vi "SubVI_SVM_Features.vi"(6 "Sigma":dbl[][](array[numeric]), 7 "MU":dbl[](array[numeric]), 8 "Scale?":bool, 9 "dt":dbl=0.05 format="%#_13g", 10 "window_time":dbl[](array[numeric]), 11 "Sliding_window":dbl[](array[numeric])) -> (1 "min value":dbl, 2 "Features_array":dbl[](array[numeric]), 3 "slope":dbl, 4 "Trap Integrate":dbl format="%0.4f", 5 "Mahibolobis":dbl)   [LabVIEW 2020]
uses:
  <vilib>/Analysis/2dsp.llb/Integral Method.ctl
  <vilib>/Analysis/8numeric.llb/1D Numeric Integration.vi
  <vilib>/Analysis/NI_AALPro.lvlib
panel:
  out "Array":dbl[][](array[numeric])
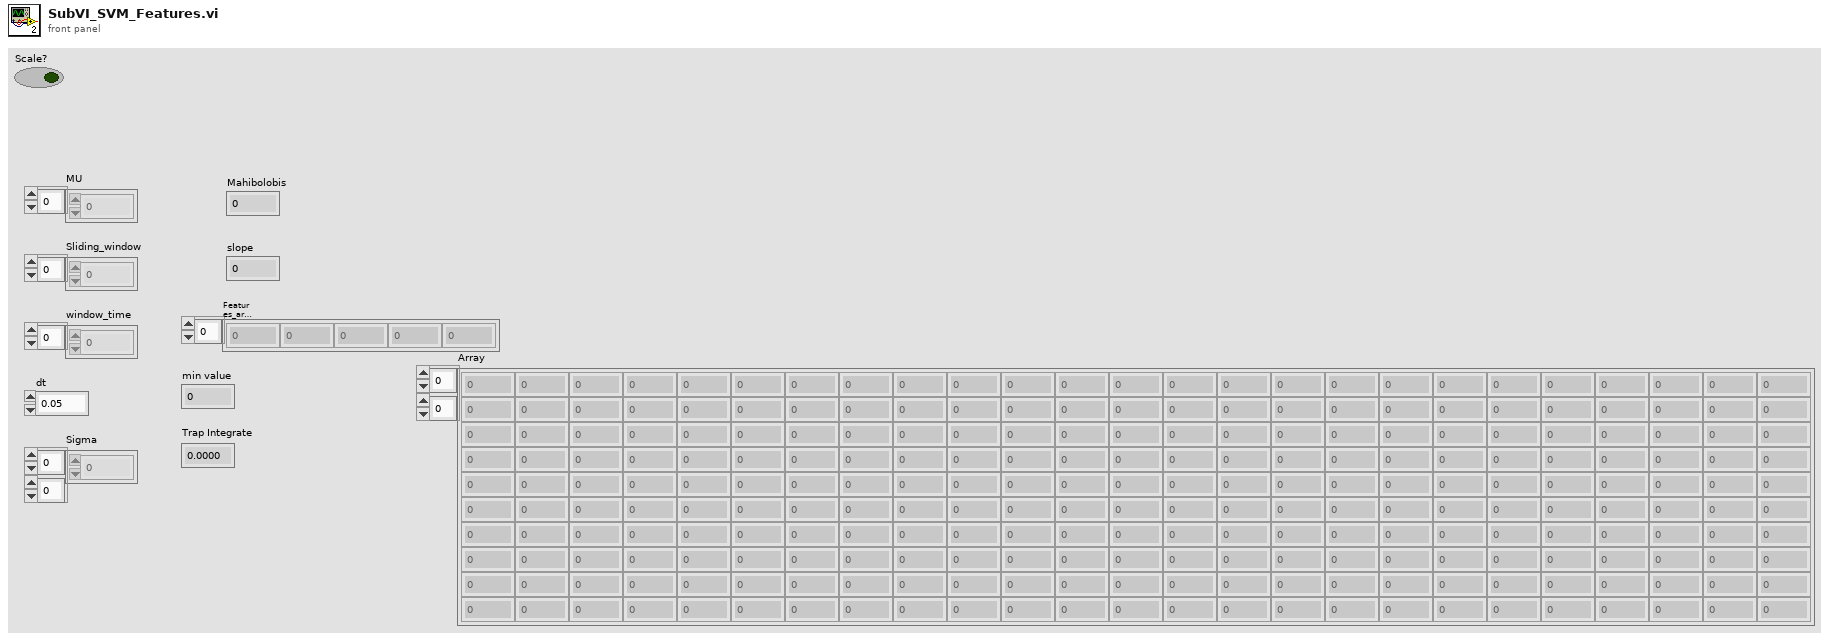
[diagram p1: front panel]
types:
  T1 = typedef "NI_AALPro.lvlib/Integral Method.ctl" = i32
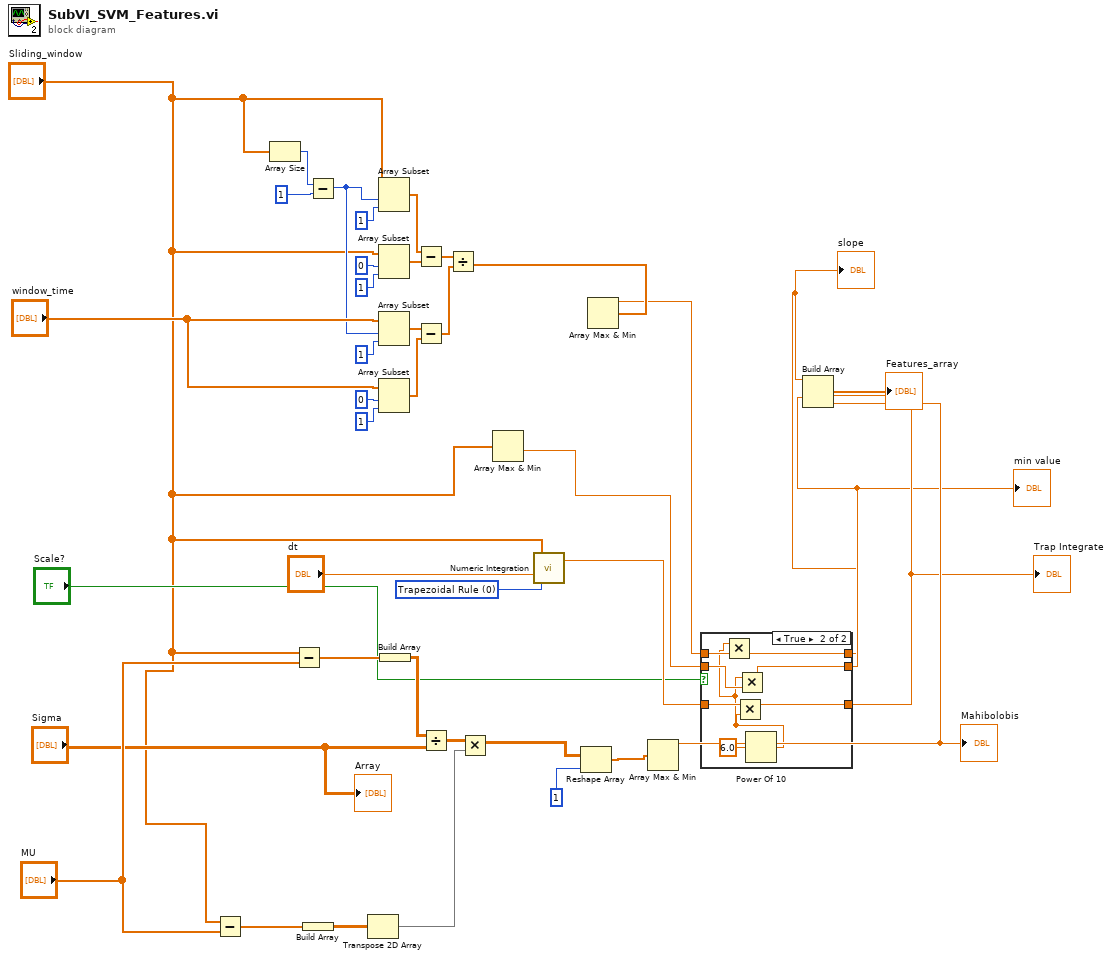
[diagram p0: block diagram]
diagram:
  w36 = T1 0 items=["Trapezoidal Rule", "Simpson's Rule", "Simpson's 3/8 Rule", "Bode Rule"] ("integration method")
  n1 = Subtract(x="Sliding_window", y="MU") -> (x-y=w32:dbl[])
  n2 = Array Size(array="Sliding_window") -> (size(s)=w15:i32)
  n3 = Subtract(x="Sliding_window", y="MU") -> (x-y=w31:dbl[])
  n4 = Build Array(w32) -> (w33:dbl[][])
  n5 = Subtract(x=w15, y=1 ("length")) -> (x-y=w13:i32)
  n6 = Transpose 2D Array(2D array=w33) -> (transposed array=w34:dbl[][])
  n7 = Array Subset(array="Sliding_window", index=w13, length=1) -> (w22:dbl[])
  n8 = Array Subset(array="Sliding_window", index=0, length=1) -> (w23:dbl[])
  n9 = Array Subset(array="window_time", index=w13, length=1) -> (w27:dbl[])
  n10 = Array Subset(array="window_time", index=0, length=1) -> (w28:dbl[])
  n11 = Build Array(w31) -> (w18:dbl[][])
  n12 = Subtract(x=w22, y=w23) -> (x-y=w29:dbl[])
  n13 = Subtract(x=w27, y=w28) -> (x-y=w30:dbl[])
  n14 = Divide(x=w18, y="Sigma") -> (x/y=w17:dbl[][])
  n15 = Divide(x=w29, y=w30) -> (x/y=w10:dbl[])
  n16 = Multiply(x=w17, y=w34) -> (x*y=w37:dbl[][])
  n17 = Array Max & Min(array="Sliding_window") -> (min value=w6:dbl)  [unwired: 3 out]
  n18 = call-poly <vilib>:"Numeric Integration.vi"("integration method"=w36, "dt"="dt", "Input Array"="Sliding_window") -> ("result"=w8:dbl)  [unwired: 1 out]
  n19 = Reshape Array(w37, 1 ("dimension size")) -> (w11:dbl[])
  n20 = Array Max & Min(array=w10) -> (max value=w4:dbl)  [unwired: 3 out]
  n21 = Array Max & Min(array=w11) -> (max value=w9:dbl)  [unwired: 3 out]
  "Mahibolobis" <- w9
  n22 = case shown="True" "Scale?" {
    tunnel: w8 -> [w41 w51]
    tunnel: [w41 w48] -> w7
    tunnel: w6 -> [w42 w50]
    tunnel: [w42 w47] -> w5
    tunnel: w4 -> [w43 w49]
    tunnel: [w43 w46] -> w3
    frame False {
    }
    frame True {
      n23 = Power Of 10(x=6.0) -> (10^x=w44:dbl)
      n24 = Multiply(x=w44, y=w49) -> (x*y=w46:dbl)
      n25 = Multiply(x=w51, y=w44) -> (x*y=w48:dbl)
      n26 = Multiply(x=w44, y=w50) -> (x*y=w47:dbl)
    }
  }
  "min value" <- w5
  "slope" <- w3
  "Trap Integrate" <- w7
  n27 = Build Array(w3, w5, w7, w9) -> (→"Features_array":dbl[])
  "Array" <- "Sigma"
